vi "20220622-InterpolateCalibration.vi"() -> ()   [LabVIEW 2016]
uses:
  <vilib>/Utility/file.llb/Read Delimited Spreadsheet (DBL).vi
  <vilib>/Utility/file.llb/Write Delimited Spreadsheet (DBL).vi
panel:
  out "transposed array":dbl[][](array[numeric])
  out "interleaved array":dbl[](array[numeric])
  in  "Tab Control 2":enum32{"Page 1", "Page 2", "Page 3", "Page 4"}(tab)
  out "2-1":dbl[][](array[numeric])=[[10.640665, 769.591383, 65.509351, -4.3e-05], [390.666052, 769.593118, 65.709351, -4.2e-05], [390.795671, 1149.618756, 65.859351, -4.2e-05], [10.772183, 1149.639611, 65.859351, -4.3e-05]]
  out "NOW1-1":dbl[][](array[numeric])=[[10.640665, 769.591383, 65.509351, -4.3e-05], [390.666052, 769.593118, 65.709351, -4.2e-05], [390.795671, 1149.618756, 65.859351, -4.2e-05], [10.772183, 1149.639611, 65.859351, -4.3e-05]]
  out "NOW2-1":dbl[][](array[numeric])=[[10.640665, 769.591383, 65.509351, -4.3e-05], [390.666052, 769.593118, 65.709351, -4.2e-05], [390.795671, 1149.618756, 65.859351, -4.2e-05], [10.772183, 1149.639611, 65.859351, -4.3e-05]]
  out "NOW2-1 減原點、距離、角度":dbl[][](array[numeric])=[[10.640665, 769.591383, 65.509351, -4.3e-05], [390.666052, 769.593118, 65.709351, -4.2e-05], [390.795671, 1149.618756, 65.859351, -4.2e-05], [10.772183, 1149.639611, 65.859351, -4.3e-05]]
  out "subarray 2":dbl[](array[numeric])
  in  "Divide":dbl[](array[numeric])=[10.640665, 769.591383, 65.509351, -4.3e-05]
  out "2-1 xy":dbl[][](array[numeric])=[[10.640665, 769.591383, 65.509351, -4.3e-05], [390.666052, 769.593118, 65.709351, -4.2e-05], [390.795671, 1149.618756, 65.859351, -4.2e-05], [10.772183, 1149.639611, 65.859351, -4.3e-05]]
  in  "Multiply":dbl[](array[numeric])=[10.640665, 769.591383, 65.509351, -4.3e-05]
  out "2-1 xy M":dbl[][](array[numeric])=[[10.640665, 769.591383, 65.509351, -4.3e-05], [390.666052, 769.593118, 65.709351, -4.2e-05], [390.795671, 1149.618756, 65.859351, -4.2e-05], [10.772183, 1149.639611, 65.859351, -4.3e-05]]
  out "2-1 xy M D":dbl[][](array[numeric])=[[10.640665, 769.591383, 65.509351, -4.3e-05], [390.666052, 769.593118, 65.709351, -4.2e-05], [390.795671, 1149.618756, 65.859351, -4.2e-05], [10.772183, 1149.639611, 65.859351, -4.3e-05]]
  out "appended array 2":dbl[][](array[numeric])
  out "2-1 d":dbl[][](array[numeric])=[[10.640665, 769.591383, 65.509351, -4.3e-05], [390.666052, 769.593118, 65.709351, -4.2e-05], [390.795671, 1149.618756, 65.859351, -4.2e-05], [10.772183, 1149.639611, 65.859351, -4.3e-05]]
  out "2-1 sub":dbl[][](array[numeric])=[[10.640665, 769.591383, 65.509351, -4.3e-05], [390.666052, 769.593118, 65.709351, -4.2e-05], [390.795671, 1149.618756, 65.859351, -4.2e-05], [10.772183, 1149.639611, 65.859351, -4.3e-05]]
  out "x/y":dbl[](array[numeric])
  out "累加array":dbl[](array[numeric])
  out "size(s)":i32[](array[numeric])
  out "累加轉置 合併2":dbl[][](array[numeric])
  out "合併1":dbl[][](array[numeric])
  out "合併後":dbl[][](array[numeric])
  in  "Tab Control":enum32{"讀取檔案", "計算結果"}(tab)
  out "X1(b)":dbl=10.640665
  out "Y1(b)":dbl=769.591376
  out "X2(b)":dbl=390.664468
  out "Y2(b)":dbl=769.591258
  out "X3 (b)":dbl=390.646567
  out "Y3 (b)":dbl=1149.621638
  out "X4 (b)":dbl=10.623763
  out "Y4 (b)":dbl=1149.646079
  out "NOW1":dbl[][](array[numeric])=[[10.640665, 769.591383, 65.509351, -4.3e-05], [390.666052, 769.593118, 65.709351, -4.2e-05], [390.795671, 1149.618756, 65.859351, -4.2e-05], [10.772183, 1149.639611, 65.859351, -4.3e-05]]
  out "NOW2":dbl[][](array[numeric])=[[10.640665, 769.591376, 65.509347, -4.2e-05], [390.664468, 769.591258, 65.759346, -4.2e-05], [390.646567, 1149.621638, 65.809344, -4.2e-05], [10.623763, 1149.646079, 65.859346, -4.2e-05]]
  out "Y2   (a)":dbl=769.593118
  out "X2  (a)":dbl=390.666052
  out "Y1   (a)":dbl=769.591383
  out "X1  (a)":dbl=10.640665
  out "X3(a)":dbl=390.795671
  out "Y3 (a)":dbl=1149.618756
  out "X4 (a)":dbl=10.772183
  out "Y4(a)":dbl=1149.639611
  out "X1":dbl
  out "Y1":dbl=-6.999999982326699e-06
  out "X2":dbl=-0.0015839999999798238
  out "X3":dbl=-0.14910400000002255
  out "X4":dbl=-0.14841999999999977
  out "Y2":dbl=-0.0018599999999651118
  out "Y4":dbl=0.0064680000000407745
  out "Y3":dbl=0.002881999999999607
  in  "目標位址座標":path=path "D:/Gantry_General/Main/ms_kao/gantry path/path data/20220616/c2 01/c2 01-1 - test/1 gantry20220616-143517.593.txt"
  in  "目前位址座標":path=path "D:/Gantry_General/Main/ms_kao/gantry path/path data/20220616/c2 01/c2 01-1 - test/2 gantry20220616-143703.227.txt"
  out "X1":dbl
  out "Y1":dbl=6.999561588732457e-06
  out "X3":dbl=-0.14909505429676473
  out "Y3":dbl=-0.0028818270903741847
  out "Y2 2":dbl=0.0018598512118681624
  out "X2":dbl=-0.0015838732901166145
  out "X4":dbl=-0.14839863840652387
  out "Y4":dbl=-0.006467069082464956
  out "12*4 2":dbl[][](array[numeric])=[[0.0, 0.0, 0.0, 0.0, 0.0, 0.0, 0.0, 0.0, 0.0, 0.0, 0.0, 0.0], [0.0, 0.0, 0.0, 0.0, 6.999561588732457e-06, 6.999561588732457e-06, -0.0015838732901166145, 0.0018598512118681624, 0.0018598512118681624, 0.0, 0.0, 0.0], [0.0, 0.0, 0.0, -0.14839863840652387, -0.006467069082464956, -0.006467069082464956, -0.14909505429676473, -0.0028818270903741847, -0.0028818270903741847, 0.0, 0.0, 0.0], [0.0, 0.0, 0.0, 0.0, 0.0, 0.0, 0.0, 0.0, 0.0, 0.0, 0.0, 0.0]]
  out "subarray":dbl[][](array[numeric])=[[0.0, 6.999561588732457e-06, 6.999561588732457e-06, -0.0015838732901166145, 0.0018598512118681624, 0.0018598512118681624], [-0.14839863840652387, -0.006467069082464956, -0.006467069082464956, -0.14909505429676473, -0.0028818270903741847, -0.0028818270903741847]]
  in  "需存取的檔案路徑":path=path "D:/Gantry_General/Main/ms_kao/gantry path/path data/20220616/c2 01/c2 01-1 - test/c2 01-1.txt"
  in  "累加偏移量 的檔案路徑":path=path "D:/Gantry_General/Main/ms_kao/gantry path/path data/20220616/c2 01/c2 01-1 - test/c2 01-1.txt"
  out "appended array":dbl[][](array[numeric])
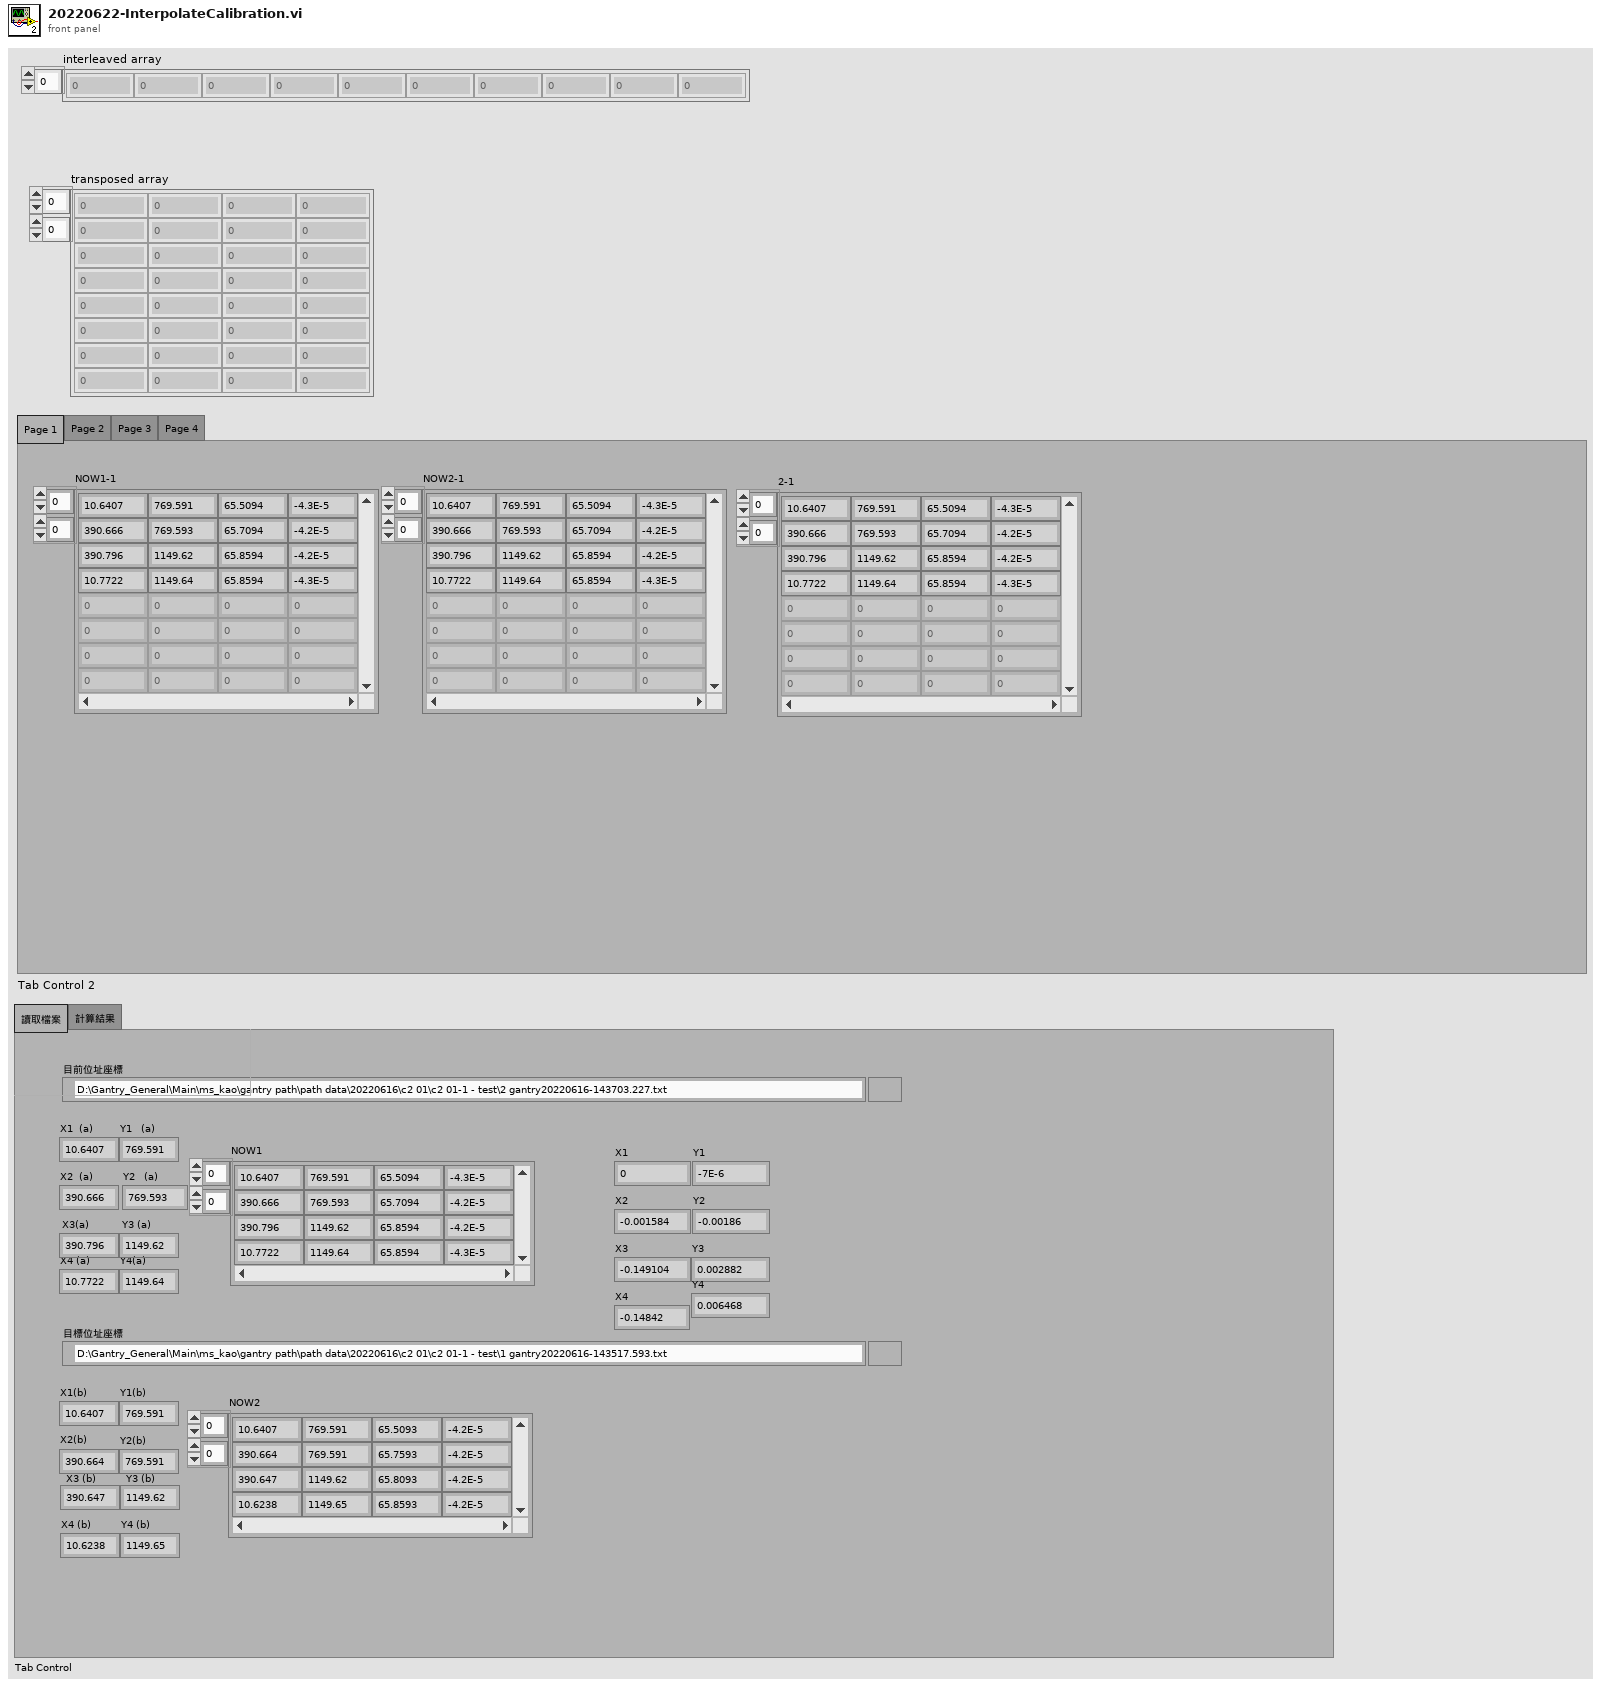
[diagram p1: front panel]
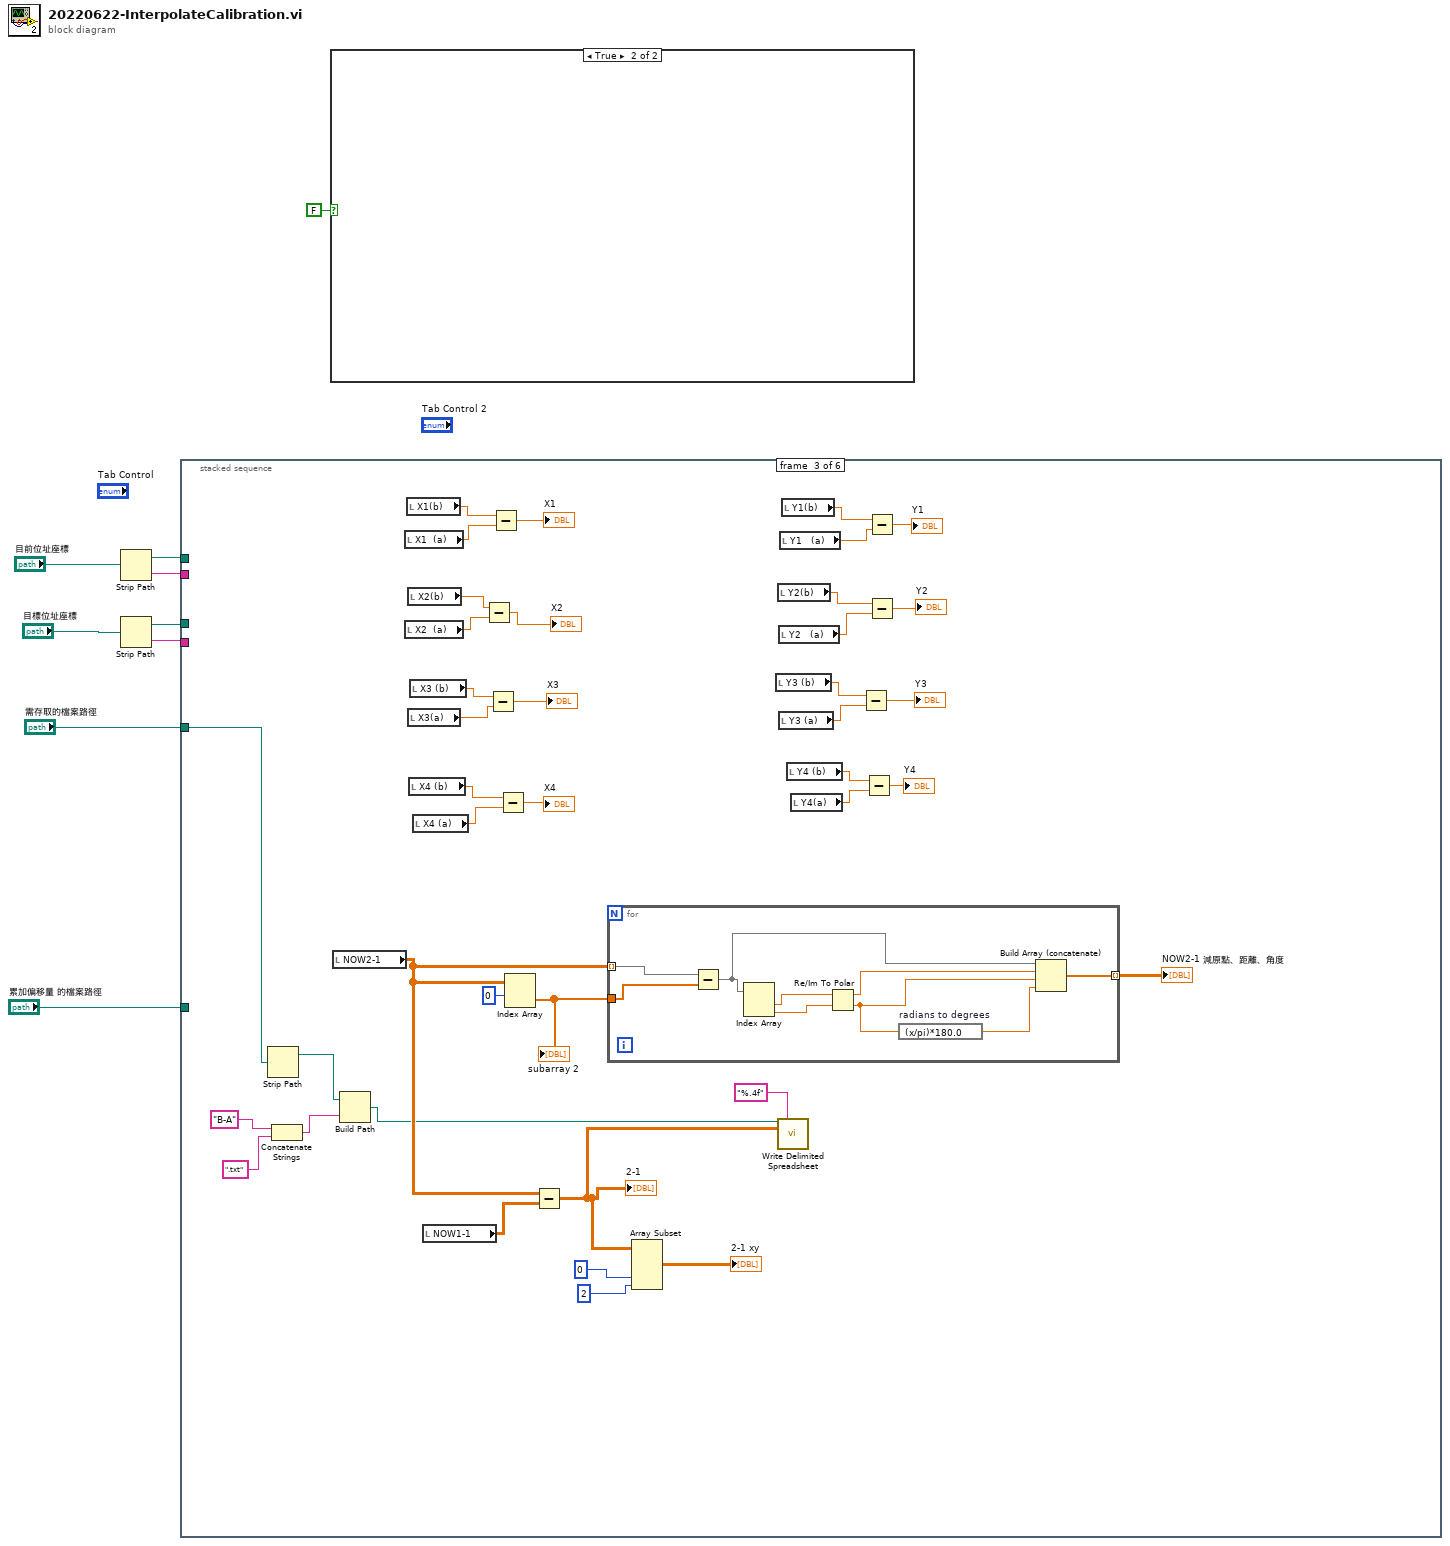
[diagram p0: block diagram]
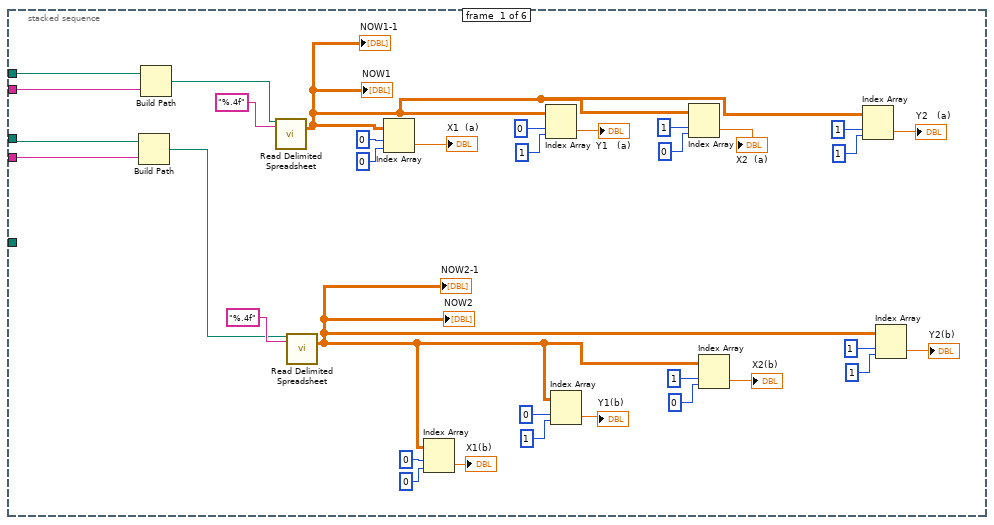
[diagram p3: hidden frame]
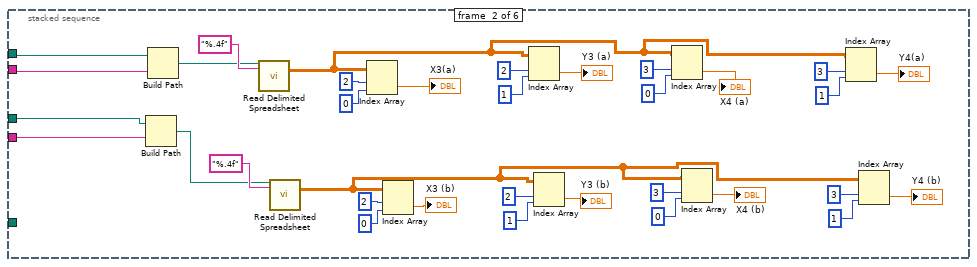
[diagram p4: hidden frame]
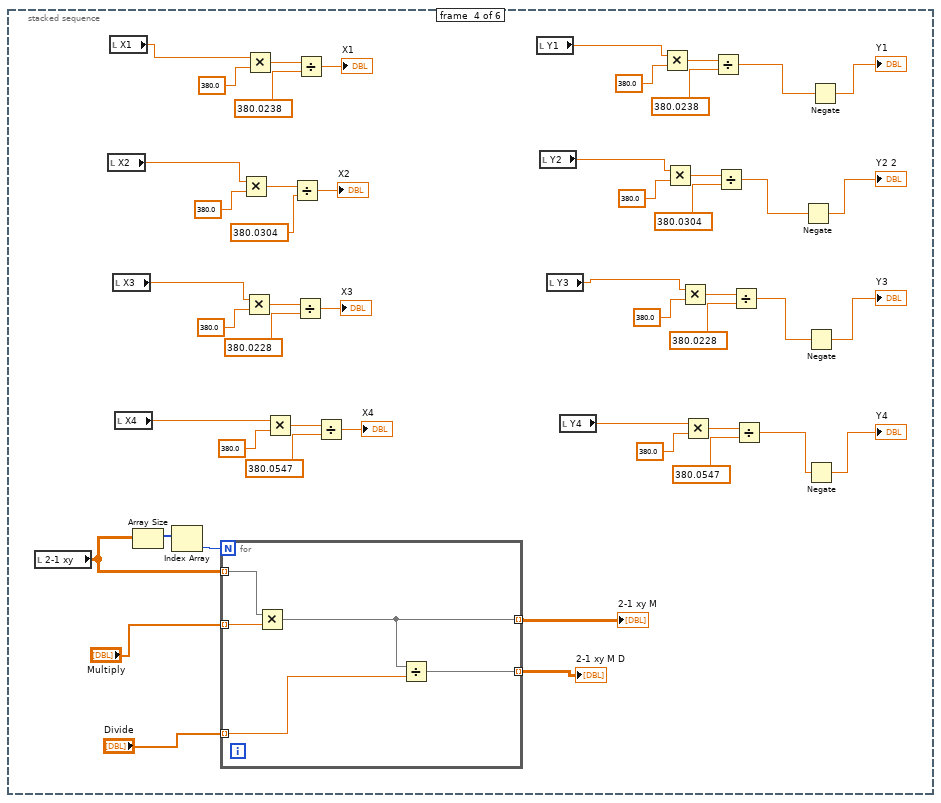
[diagram p5: hidden frame]
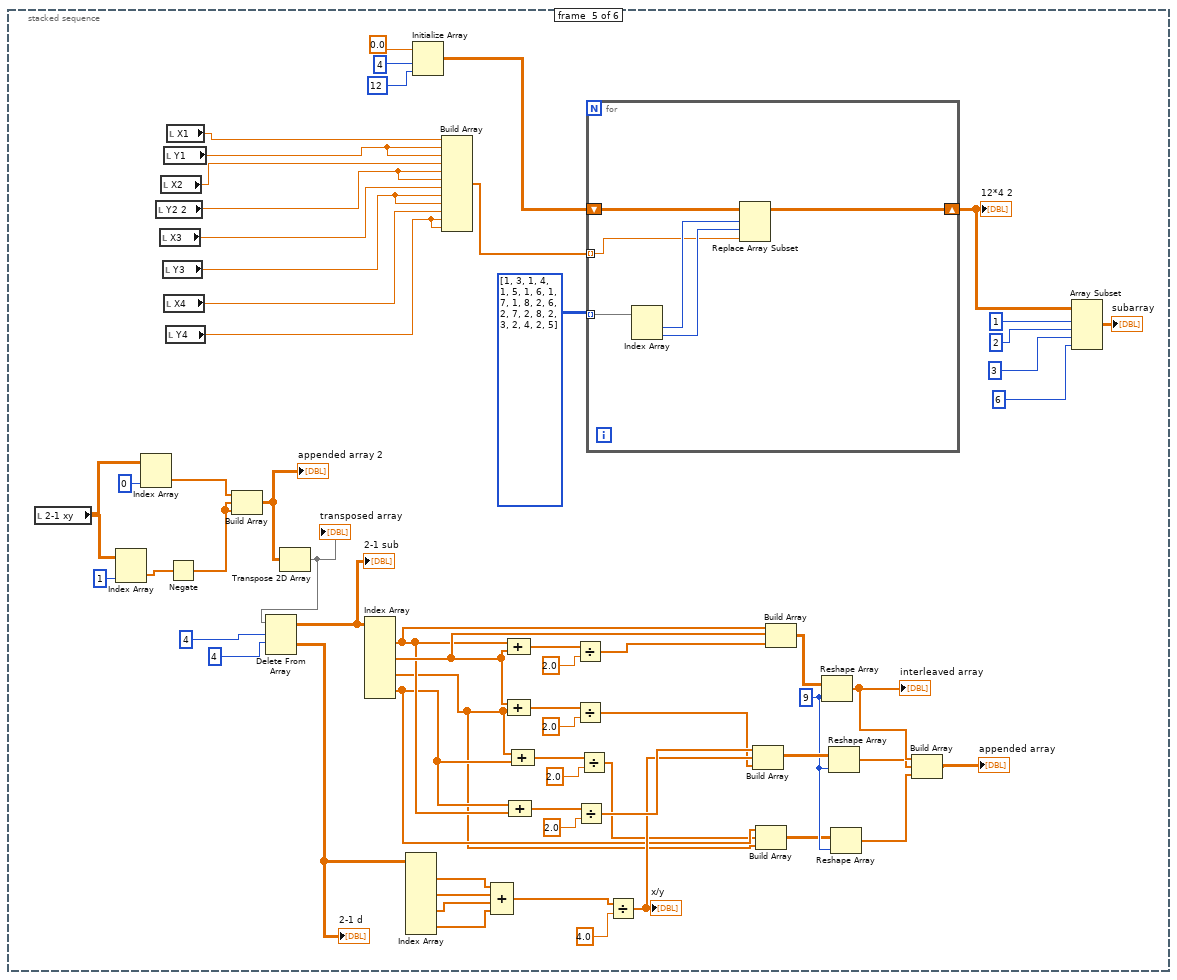
[diagram p6: hidden frame]
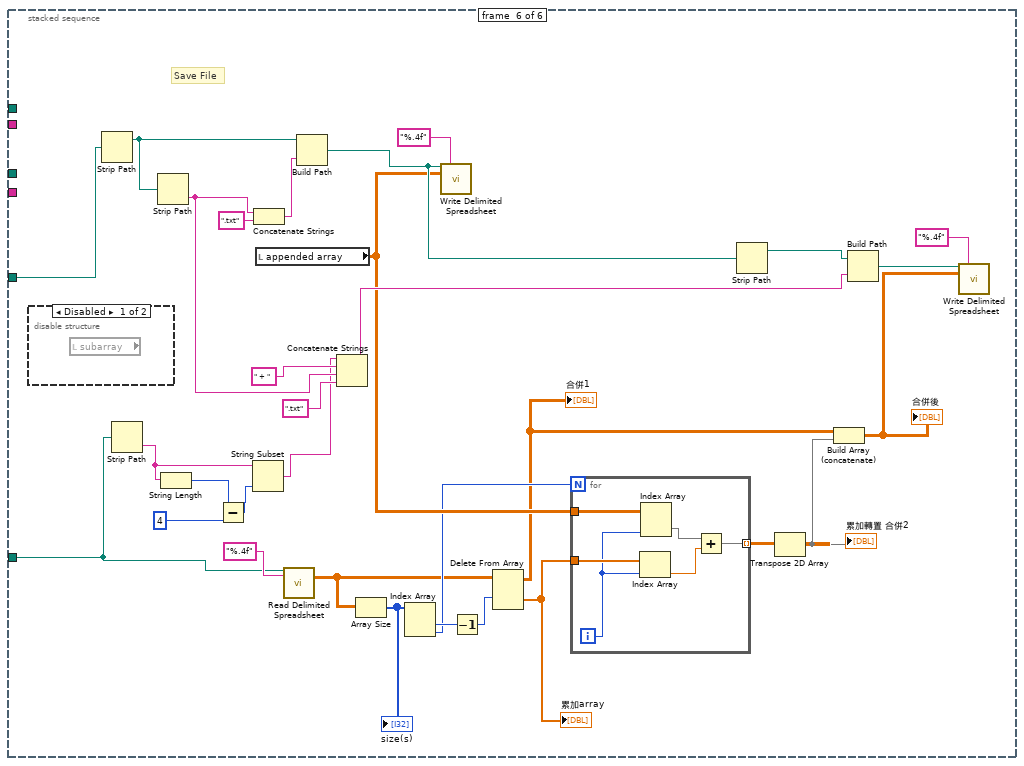
[diagram p7: hidden frame]
diagram:
  n1 = Strip Path(path="目前位址座標") -> (stripped path=w9:path, name=w8:string)
  n2 = Strip Path(path="目標位址座標") -> (stripped path=w7:path, name=w6:string)
  n3 = stacked-sequence {
    tunnel: w9 -> [w39 w44 _ _ _ _]
    tunnel: w8 -> [w37 w45 _ _ _ _]
    tunnel: w7 -> [w36 w46 _ _ _ _]
    tunnel: w6 -> [w35 w47 _ _ _ _]
    tunnel: "需存取的檔案路徑" -> [_ _ w84 _ _ w253]
    tunnel: "累加偏移量 的檔案路徑" -> [_ _ _ _ _ w252]
    frame #0 {
      n4 = Build Path(base path=w36, name or relative path=w35) -> (appended path=w30:path)
      n5 = Build Path(base path=w39, name or relative path=w37) -> (appended path=w38:path)
      n6 = call-poly <vilib>:"Read Delimited Spreadsheet.vi"("file path (dialog if empty)"=w38, "format (%.3f)"="%.4f") -> ("all rows"=w11:dbl[][])  [unwired: 8 in, 5 out]
      "NOW1" <- w11
      "NOW1-1" <- w11
      n7 = call-poly <vilib>:"Read Delimited Spreadsheet.vi"("file path (dialog if empty)"=w30, "format (%.3f)"="%.4f") -> ("all rows"=w10:dbl[][])  [unwired: 8 in, 5 out]
      "NOW2" <- w10
      "NOW2-1" <- w10
      n8 = Index Array(array=w11, index (row)=0, index (col)=0 ("disabled index (col)")) -> (element=→"X1  (a)":dbl)
      n9 = Index Array(array=w10, index (row)=0, index (col)=0 ("disabled index (col)")) -> (element=→"X1(b)":dbl)
      n10 = Index Array(array=w11, index (row)=0, index (col)=1 ("disabled index (col)")) -> (element=→"Y1   (a)":dbl)
      n11 = Index Array(array=w10, index (row)=0, index (col)=1 ("disabled index (col)")) -> (element=→"Y1(b)":dbl)
      n12 = Index Array(array=w11, index (row)=1, index (col)=0 ("disabled index (col)")) -> (element=→"X2  (a)":dbl)
      n13 = Index Array(array=w10, index (row)=1, index (col)=0 ("disabled index (col)")) -> (element=→"X2(b)":dbl)
      n14 = Index Array(array=w11, index (row)=1, index (col)=1 ("disabled index (col)")) -> (element=→"Y2   (a)":dbl)
      n15 = Index Array(array=w10, index (row)=1, index (col)=1 ("disabled index (col)")) -> (element=→"Y2(b)":dbl)
    }
    frame #1 {
      n16 = Build Path(base path=w46, name or relative path=w47) -> (appended path=w68:path)
      n17 = Build Path(base path=w44, name or relative path=w45) -> (appended path=w73:path)
      n18 = call-poly <vilib>:"Read Delimited Spreadsheet.vi"("file path (dialog if empty)"=w73, "format (%.3f)"="%.4f") -> ("all rows"=w48:dbl[][])  [unwired: 8 in, 5 out]
      n19 = call-poly <vilib>:"Read Delimited Spreadsheet.vi"("file path (dialog if empty)"=w68, "format (%.3f)"="%.4f") -> ("all rows"=w52:dbl[][])  [unwired: 8 in, 5 out]
      n20 = Index Array(array=w48, index (row)=2, index (col)=0 ("disabled index (col)")) -> (element=→"X3(a)":dbl)
      n21 = Index Array(array=w52, index (row)=2, index (col)=0 ("disabled index (col)")) -> (element=→"X3 (b)":dbl)
      n22 = Index Array(array=w48, index (row)=2, index (col)=1 ("disabled index (col)")) -> (element=→"Y3 (a)":dbl)
      n23 = Index Array(array=w52, index (row)=2, index (col)=1 ("disabled index (col)")) -> (element=→"Y3 (b)":dbl)
      n24 = Index Array(array=w48, index (row)=3, index (col)=0 ("disabled index (col)")) -> (element=→"X4 (a)":dbl)
      n25 = Index Array(array=w52, index (row)=3, index (col)=0 ("disabled index (col)")) -> (element=→"X4 (b)":dbl)
      n26 = Index Array(array=w48, index (row)=3, index (col)=1 ("disabled index (col)")) -> (element=→"Y4(a)":dbl)
      n27 = Index Array(array=w52, index (row)=3, index (col)=1 ("disabled index (col)")) -> (element=→"Y4 (b)":dbl)
    }
    frame #2 {
      n28 = Strip Path(path=w84) -> (stripped path=w83:path)  [unwired: 1 out]
      n29 = Concatenate Strings("B-A" ("string"), ".txt" ("string")) -> (w80:string)
      n30 = local read "NOW2-1"() -> (w89:dbl[][])
      n31 = Build Path(base path=w83, name or relative path=w80) -> (appended path=w79:path)
      n32 = local read "X1  (a)"() -> (w116:dbl)
      n33 = local read "X2  (a)"() -> (w113:dbl)
      n34 = local read "X1(b)"() -> (w117:dbl)
      n35 = local read "X2(b)"() -> (w112:dbl)
      n36 = local read "X3(a)"() -> (w110:dbl)
      n37 = local read "X4 (b)"() -> (w105:dbl)
      n38 = local read "X3 (b)"() -> (w111:dbl)
      n39 = local read "X4 (a)"() -> (w104:dbl)
      n40 = local read "NOW1-1"() -> (w93:dbl[][])
      n41 = Subtract(x=w112, y=w113) -> (x-y=→"X2":dbl)
      n42 = Subtract(x=w111, y=w110) -> (x-y=→"X3":dbl)
      n43 = Subtract(x=w117, y=w116) -> (x-y=→"X1":dbl)
      n44 = Subtract(x=w105, y=w104) -> (x-y=→"X4":dbl)
      n45 = Index Array(array=w89, index (row)=0) -> (element=w87:dbl[])  [unwired: 1 in]
      "subarray 2" <- w87
      n46 = Subtract(x=w89, y=w93) -> (x-y=w78:dbl[][])
      "2-1" <- w78
      n47 = for {
        tunnel: w89 -> [w126] mode=indexing
        tunnel: w87 -> [w125]
        tunnel: [w120] -> w86 mode=indexing
        n48 = Subtract(x=w126, y=w125) -> (x-y=w121:dbl[])
        n49 = Index Array(array=w121) -> (element #1=w124:dbl, element #2=w123:dbl)  [unwired: 2 in]
        n50 = Re/Im To Polar(2:w123, 3:w124) -> (0:w118:dbl, 1:w122:dbl)
        n51 = expression code="(x/pi)*180.0" "radians to degrees"(w118) -> (w119:dbl)
        n52 = Build Array (concatenate)(w121, w122, w118, w119) -> (w120:dbl[])
      }
      "NOW2-1 減原點、距離、角度" <- w86
      n53 = Array Subset(array=w78, index (col)=0 ("index"), length (col)=2 ("length")) -> (→"2-1 xy":dbl[][])  [unwired: 2 in]
      n54 = local read "Y3 (b)"() -> (w107:dbl)
      n55 = local read "Y2(b)"() -> (w103:dbl)
      n56 = call-poly <vilib>:"Write Delimited Spreadsheet.vi"("file path (dialog if empty)"=w79, "format (%.3f)"="%.4f", "2D data"=w78) -> ()  [unwired: 11 in, 2 out]
      n57 = local read "Y2   (a)"() -> (w102:dbl)
      n58 = local read "Y3 (a)"() -> (w106:dbl)
      n59 = local read "Y1   (a)"() -> (w114:dbl)
      n60 = local read "Y1(b)"() -> (w115:dbl)
      n61 = local read "Y4 (b)"() -> (w109:dbl)
      n62 = local read "Y4(a)"() -> (w108:dbl)
      n63 = Subtract(x=w107, y=w106) -> (x-y=→"Y3":dbl)
      n64 = Subtract(x=w109, y=w108) -> (x-y=→"Y4":dbl)
      n65 = Subtract(x=w115, y=w114) -> (x-y=→"Y1":dbl)
      n66 = Subtract(x=w103, y=w102) -> (x-y=→"Y2":dbl)
    }
    frame #3 {
      n67 = local read "2-1 xy"() -> (w133:dbl[][])
      n68 = local read "X2"() -> (w148:dbl)
      n69 = local read "X1"() -> (w149:dbl)
      n70 = local read "X3"() -> (w144:dbl)
      n71 = local read "X4"() -> (w143:dbl)
      n72 = Array Size(array=w133) -> (size(s)=w132:i32[])
      n73 = Index Array(array=w132) -> (element=w131:i32)  [unwired: 1 in]
      n74 = for {
        N: w131 -> [_]
        tunnel: w133 -> [w182] mode=indexing
        tunnel: "Multiply" -> [w181] mode=indexing
        tunnel: "Divide" -> [w180] mode=indexing
        tunnel: [w179] -> w127 mode=indexing
        tunnel: [w178] -> w128 mode=indexing
        n75 = Multiply(x=w182, y=w181) -> (x*y=w178:dbl[])
        n76 = Divide(x=w178, y=w180) -> (x/y=w179:dbl[])
      }
      "2-1 xy M D" <- w127
      "2-1 xy M" <- w128
      n77 = Multiply(x=w148, y=380.0) -> (x*y=w164:dbl)
      n78 = Multiply(x=w144, y=380.0) -> (x*y=w162:dbl)
      n79 = Multiply(x=w149, y=380.0) -> (x*y=w167:dbl)
      n80 = Multiply(x=w143, y=380.0) -> (x*y=w158:dbl)
      n81 = Divide(x=w164, y=380.0304) -> (x/y=→"X2":dbl)
      n82 = Divide(x=w162, y=380.0228) -> (x/y=→"X3":dbl)
      n83 = Divide(x=w167, y=380.0238) -> (x/y=→"X1":dbl)
      n84 = Divide(x=w158, y=380.0547) -> (x/y=→"X4":dbl)
      n85 = local read "Y1"() -> (w147:dbl)
      n86 = local read "Y2"() -> (w146:dbl)
      n87 = local read "Y3"() -> (w145:dbl)
      n88 = local read "Y4"() -> (w142:dbl)
      n89 = Multiply(x=w147, y=380.0) -> (x*y=w176:dbl)
      n90 = Multiply(x=w146, y=380.0) -> (x*y=w173:dbl)
      n91 = Multiply(x=w145, y=380.0) -> (x*y=w170:dbl)
      n92 = Multiply(x=w142, y=380.0) -> (x*y=w155:dbl)
      n93 = Divide(x=w176, y=380.0238) -> (x/y=w141:dbl)
      n94 = Divide(x=w173, y=380.0304) -> (x/y=w135:dbl)
      n95 = Divide(x=w170, y=380.0228) -> (x/y=w137:dbl)
      n96 = Divide(x=w155, y=380.0547) -> (x/y=w139:dbl)
      n97 = Negate(x=w135) -> (-x=→"Y2 2":dbl)
      n98 = Negate(x=w137) -> (-x=→"Y3":dbl)
      n99 = Negate(x=w139) -> (-x=→"Y4":dbl)
      n100 = Negate(x=w141) -> (-x=→"Y1":dbl)
    }
    frame #4 {
      w198 = 9 ("dimension size")
      n101 = local read "2-1 xy"() -> (w189:dbl[][])
      n102 = Index Array(array=w189, index (col)=1 ("disabled index (col)")) -> (element=w187:dbl[])  [unwired: 1 in]
      n103 = Index Array(array=w189, index (col)=0 ("disabled index (col)")) -> (element=w186:dbl[])  [unwired: 1 in]
      n104 = local read "Y2 2"() -> (w239:dbl)
      n105 = local read "X3"() -> (w238:dbl)
      n106 = local read "X2"() -> (w240:dbl)
      n107 = local read "Y3"() -> (w237:dbl)
      n108 = local read "Y1"() -> (w241:dbl)
      n109 = local read "X4"() -> (w236:dbl)
      n110 = local read "Y4"() -> (w235:dbl)
      n111 = local read "X1"() -> (w242:dbl)
      n112 = Negate(x=w187) -> (-x=w185:dbl[])
      n113 = Build Array(w186, w185, w185) -> (w184:dbl[][])
      "appended array 2" <- w184
      n114 = Transpose 2D Array(2D array=w184) -> (transposed array=w183:dbl[][])
      "transposed array" <- w183
      n115 = Delete From Array(array=w183, length=4, index (row)=4 ("disabled index (col)")) -> (deleted portion=w221:dbl[][], array with subset deleted=w222:dbl[][])  [unwired: 1 in]
      "2-1 sub" <- w222
      "2-1 d" <- w221
      n116 = Index Array(array=w222) -> (element #1=w205:dbl[], element #2=w206:dbl[], element #3=w195:dbl[], element #4=w197:dbl[])  [unwired: 8 in]
      n117 = Index Array(array=w221) -> (element #1=w220:dbl[], element #2=w219:dbl[], element #3=w218:dbl[], element #4=w217:dbl[])  [unwired: 8 in]
      n118 = Initialize Array(0.0 ("element"), 4 ("dimension size"), 12 ("dimension size")) -> (w232:dbl[][])
      n119 = Build Array(w242, w241, w241, w240, w239, w239, w238, w237, w237, w236, w235, w235) -> (w234:dbl[])
      n120 = Compound Arithmetic op=ADD(w220, w219, w218, w217) -> (w216:dbl[])
      n121 = Compound Arithmetic op=ADD(w205, w206) -> (w215:dbl[])
      n122 = Compound Arithmetic op=ADD(w206, w195) -> (w212:dbl[])
      n123 = Compound Arithmetic op=ADD(w197, w205) -> (w211:dbl[])
      n124 = Compound Arithmetic op=ADD(w195, w197) -> (w208:dbl[])
      n125 = Divide(x=w215, y=2.0) -> (x/y=w204:dbl[])
      n126 = Divide(x=w212, y=2.0) -> (x/y=w200:dbl[])
      n127 = Divide(x=w211, y=2.0) -> (x/y=w202:dbl[])
      n128 = Divide(x=w208, y=2.0) -> (x/y=w196:dbl[])
      n129 = for {
        tunnel: w234 -> [w247] mode=indexing
        tunnel: i32[][] [[1, 3], [1, 4], [1, 5], [1, 6], [1, 7], [1, 8], [2, 6], [2, 7], [2, 8], [2, 3], [2, 4], [2, 5]] -> [w251] mode=indexing
        shift-right: [w246] -> w231
        shift-left: w232 -> [w250]
        n130 = Index Array "Index Array"(array=w251) -> (element #1=w249:i32, element #2=w248:i32)  [unwired: 2 in]
        n131 = Replace Array Subset "Replace Array Subset"(array=w250, new element=w247, index (row)=w249, index (col)=w248) -> (w246:dbl[][])
      }
      "12*4 2" <- w231
      n132 = Divide(x=w216, y=4.0) -> (x/y=w201:dbl[])
      "x/y" <- w201
      n133 = Build Array(w202, w201, w200) -> (w199:dbl[][])
      n134 = Build Array(w197, w196, w195) -> (w194:dbl[][])
      n135 = Build Array(w205, w204, w206) -> (w203:dbl[][])
      n136 = Reshape Array(w203, w198) -> (w193:dbl[])
      "interleaved array" <- w193
      n137 = Reshape Array(w199, w198) -> (w192:dbl[])
      n138 = Reshape Array(w194, w198) -> (w191:dbl[])
      n139 = Build Array(w193, w192, w191) -> (→"appended array":dbl[][])
      n140 = Array Subset(array=w231, index (row)=1 ("index"), length (row)=2 ("index"), index (col)=3 ("index"), length (col)=6 ("index")) -> (→"subarray":dbl[][])
    }
    frame #5 {
      # "Save File"
      n141 = disable-structure shown="Disabled" {
        frame Disabled {
          n142 = local read "subarray"() -> ()  [unwired: 1 out]
        }
        frame Enabled {
        }
      }
      n143 = Strip Path(path=w253) -> (stripped path=w275:path)  [unwired: 1 out]
      n144 = Strip Path(path=w252) -> (name=w256:string)  [unwired: 1 out]
      n145 = Strip Path(path=w275) -> (name=w259:string)  [unwired: 1 out]
      n146 = String Length(string=w256) -> (length=w258:i32)
      n147 = Subtract(x=w258, y=4) -> (x-y=w254:i32)
      n148 = String Subset(string=w256, length (rest)=w254) -> (substring=w255:string)  [unwired: 1 in]
      n149 = Concatenate Strings(w259, ".txt" ("string")) -> (w274:string)
      n150 = local read "appended array"() -> (w269:dbl[][])
      n151 = call-poly <vilib>:"Read Delimited Spreadsheet.vi"("file path (dialog if empty)"=w252, "format (%.3f)"="%.4f") -> ("all rows"=w266:dbl[][])  [unwired: 8 in, 5 out]
      n152 = Build Path(base path=w275, name or relative path=w274) -> (appended path=w276:path)
      n153 = Concatenate Strings(w255, " + " ("name or relative path"), w259, ".txt" ("string")) -> (w272:string)
      n154 = Array Size(array=w266) -> (size(s)=w271:i32[])
      "size(s)" <- w271
      n155 = Index Array(array=w271) -> (element #1=w270:i32, element #2=w267:i32)  [unwired: 2 in]
      n156 = call-poly <vilib>:"Write Delimited Spreadsheet.vi"("file path (dialog if empty)"=w276, "format (%.3f)"="%.4f", "2D data"=w269) -> ()  [unwired: 11 in, 2 out]
      n157 = Decrement(x=w270) -> (x-1=w265:i32)
      n158 = Delete From Array(array=w266, index (row)=w265) -> (deleted portion=w264:dbl[], array with subset deleted=w262:dbl[][])  [unwired: 2 in]
      "累加array" <- w264
      "合併1" <- w262
      n159 = for {
        N: w267 -> [_]
        tunnel: w269 -> [w288]
        tunnel: w264 -> [w287]
        tunnel: [w283] -> w268 mode=indexing
        i -> [w286]
        n160 = Index Array(array=w287, index=w286) -> (element=w284:dbl)
        n161 = Index Array(array=w288, index (col)=w286) -> (element=w285:dbl[])  [unwired: 1 in]
        n162 = Add(x=w285, y=w284) -> (x+y=w283:dbl[])
      }
      n163 = Strip Path(path=w276) -> (stripped path=w279:path)  [unwired: 1 out]
      n164 = Transpose 2D Array(2D array=w268) -> (transposed array=w263:dbl[][])
      "累加轉置 合併2" <- w263
      n165 = Build Array (concatenate)(w262, w263) -> (w261:dbl[][])
      "合併後" <- w261
      n166 = Build Path(base path=w279, name or relative path=w272) -> (appended path=w278:path)
      n167 = call-poly <vilib>:"Write Delimited Spreadsheet.vi"("file path (dialog if empty)"=w278, "format (%.3f)"="%.4f", "2D data"=w261) -> ()  [unwired: 11 in, 2 out]
    }
  }
  n168 = case shown="True" FALSE {
    frame False {
    }
    frame True {
    }
  }
